vi "Update LV Class Version.vi"(11 "LV Class File Path":string="ModifiedClass.lvclass") -> (0 "error out":errorcluster)   [LabVIEW 2012]
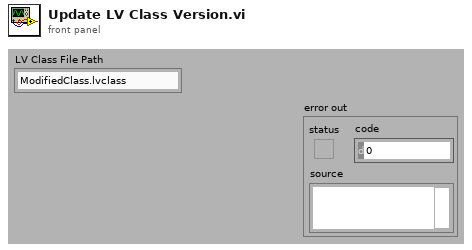
[diagram p1: front panel]
types:
  T1 = cluster{"Major":u16, "Minor":u16, "Fix":u16, "Build":u16}
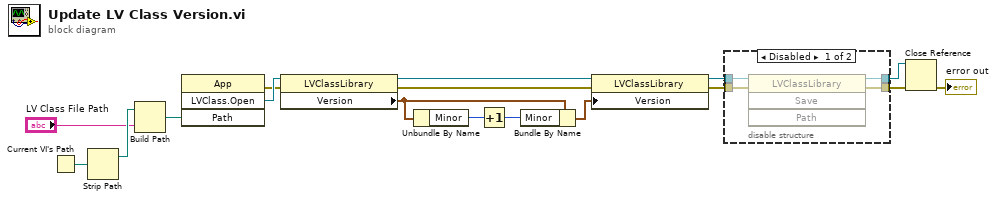
[diagram p0: block diagram]
diagram:
  n1 = Current VI's Path() -> (path=w17:path)
  n2 = Strip Path(path=w17) -> (stripped path=w16:path)  [unwired: 1 out]
  n3 = Build Path(base path=w16, name or relative path="LV Class File Path") -> (appended path=w14:path)
  n4 = invoke class="App" method="LVClass.Open"("Path"=w14) -> (error out=w12:errorcluster, "LVClass.Open"=w13:refnum<vi>)  [unwired: 3 in, 2 out]
  n5 = property class="LVClassLibrary"(reference=w13, error in=w12) -> (reference out=w8:refnum<vi>, error out=w7:errorcluster, "Version"=w9:T1)
  n6 = Unbundle By Name(w9) -> ("Minor"=w11:u16)
  n7 = Increment(x=w11) -> (x+1=w10:u16)
  n8 = Bundle By Name(cluster=w9, "Minor"=w10) -> (w6:T1)
  n9 = property class="LVClassLibrary"(reference=w8, error in=w7, "Version"=w6) -> (reference out=w5:refnum<vi>, error out=w4:errorcluster)
  n10 = disable-structure shown="Disabled" {
    disable-tunnel: w5 -> [w21 w23]
    disable-tunnel: w4 -> [w20 w22]
    disable-tunnel: [w19 w22] -> w3
    disable-tunnel: [w18 w23] -> w2
    frame Disabled {
      n11 = invoke class="LVClassLibrary" method="Save"(reference=w21, error in=w20) -> (reference out=w18:refnum<vi>, error out=w19:errorcluster)  [unwired: 2 in, 2 out]
    }
    frame Enabled {
    }
  }
  n12 = Close Reference(reference=w2, error in (no error)=w3) -> (error out=→"error out":errorcluster)
